vi "2 Tap 10-Bit.vi"() -> (0 "Pixels":cluster{"Pixel 0":u16, "Pixel 1":u16})   [LabVIEW 2013]
uses:
  <vilib>/rvi/eio/common/nirviEmuTemplateMethod_errors.vi
  <vilib>/eio/EIONode/EIONode.xnode
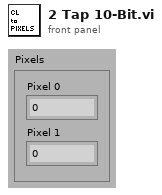
[diagram p1: front panel]
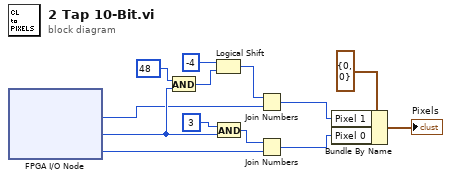
[diagram p0: block diagram]
diagram:
  n1 = xnode "FPGA I/O Node"() -> ("CL Port C"=w3:u8, "CL Port B"=w5:u8, "CL Port A"=w4:u8)  [unwired: 3 in, 3 out]
  n2 = And(x=u8 48 ("hi"), y=w5) -> (x .and. y?=w8:u8)
  n3 = Logical Shift(y=i8 -4, x=w8) -> (x << y=w6:u8)
  n4 = And(x=u8 3 ("hi"), y=w5) -> (x .and. y?=w10:u8)
  n5 = Join Numbers(hi=w6, lo=w3) -> ((hi.lo)=w1:u16)
  n6 = Join Numbers(hi=w10, lo=w4) -> ((hi.lo)=w2:u16)
  n7 = Bundle By Name(cluster=cluster{"Pixel 0":u16, "Pixel 1":u16} {"Pixel 0"=0, "Pixel 1"=0} ("PixelData"), "Pixel 1"=w1, "Pixel 0"=w2) -> (→"Pixels":cluster{"Pixel 0":u16, "Pixel 1":u16})
